vi "NML SCMPS make persistent.vi"(0 "VISA session":refnum<visa-resource-name>="GPIB0::22::INSTR") -> (2 "String":string, 3 "Persistent Field":dbl format="%.2f", 4 "Persistence Out":bool=TRUE)   [LabVIEW 2020]
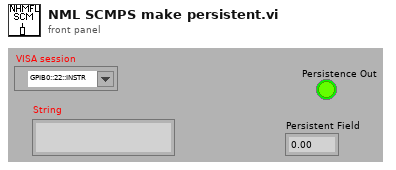
[diagram p1: front panel]
types:
  T1 = enum16{"No Response", "Ramping to programmed field ", "Holding at programmed field", "Paused", "Ramp Manual Up", "Ramp Manual Down", "Ramping to Zero", "QUENCH", "Heating Persistence Switch", "At Zero Current"}
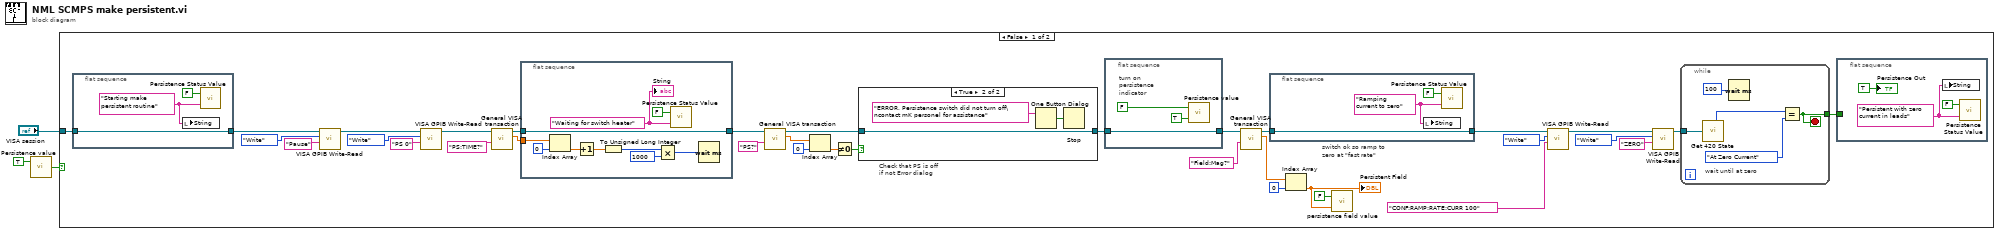
[diagram p0: block diagram]
diagram:
  n1 = call "Persistence value.vi"("Read/Write this vi"=TRUE ("Read/Write")) -> ("Persistence Out"=w2:bool)  [unwired: 1 in]
  n2 = case shown="False" w2 {
    tunnel: "VISA session" -> [w5 _]
    frame False {
      # "Check that PS is off \nif not Error dialog"
      # "switch ok so ramp to zero at \"fast rate\""
      n3 = flat-sequence {
        tunnel: w5 -> [w38]
        tunnel: [w38] -> w4
        frame #0 {
          w39 = "Starting make persistent routine"
          n4 = local write "String"(w39) -> ()
          n5 = call "Persistence Status Value.vi"("Persistence Status In"=w39, "Read/Write this vi"=FALSE) -> ()  [unwired: 1 out]
        }
      }
      n6 = call "VISA GPIB Write-Read.vi"("Command"="Pause" ("String to Write"), "Action"=enum16{"Write", "Read", "Write & Read"}."Write", "VISA resource name"=w4) -> ("dup VISA Session"=w12:refnum<visa-resource-name>)  [unwired: 5 in, 3 out]
      n7 = call "VISA GPIB Write-Read.vi"("Command"="PS 0" ("String to Write"), "Action"=enum16{"Write", "Read", "Write & Read"}."Write", "VISA resource name"=w12) -> ("dup VISA Session"=w17:refnum<visa-resource-name>)  [unwired: 5 in, 3 out]
      n8 = call "General VISA transaction.vi"("Command String"="PS:TIME?", "VISA Session"=w17) -> ("Measurement"=w15:dbl[], "dup VISA Session"=w16:refnum<visa-resource-name>)  [unwired: 4 in, 4 out]
      n9 = flat-sequence {
        tunnel: w16 -> [w41]
        tunnel: w15 -> [w42]
        tunnel: [w41] -> w19
        frame #0 {
          w50 = "Waiting for switch heater"
          n10 = Index Array(array=w42, index=0) -> (element=w45:dbl)
          n11 = Increment(x=w45) -> (x+1=w47:dbl)
          n12 = To Unsigned Long Integer(number=w47) -> (unsigned 32bit integer=w48:u32)
          n13 = Multiply(x=w48, y=u32 1000) -> (x*y=w46:u32)
          n14 = call "Persistence Status Value.vi"("Persistence Status In"=w50, "Read/Write this vi"=FALSE) -> ()  [unwired: 1 out]
          n15 = Wait (ms)(milliseconds to wait=w46) -> ()  [unwired: 1 out]
          "String" <- w50
        }
      }
      n16 = call "General VISA transaction.vi"("Command String"="PS?", "VISA Session"=w19) -> ("Measurement"=w24:dbl[], "dup VISA Session"=w20:refnum<visa-resource-name>)  [unwired: 4 in, 4 out]
      n17 = Index Array(array=w24, index=0) -> (element=w22:dbl)
      n18 = Not Equal To 0?(x=w22) -> (x != 0?=w21:bool)
      n19 = case shown="True" w21 {
        tunnel: w20 -> [w54 w55]
        tunnel: [w54 w55] -> w7
        frame False {
        }
        frame True {
          n20 = One Button Dialog(message="ERROR, Persistence switch did not turn off\ncontact mK personel for assistance") -> (true=w56:bool)  [unwired: 1 in]
          n21 = Stop(stop? (T)=w56) -> ()
        }
      }
      n22 = flat-sequence {
        tunnel: w7 -> [w51]
        tunnel: [w51] -> w6
        frame #0 {
          # "turn on persistence indicator"
          n23 = call "Persistence value.vi"("Persistence In"=TRUE, "Read/Write this vi"=FALSE) -> ()  [unwired: 1 out]
        }
      }
      n24 = call "General VISA transaction.vi"("Command String"="Field:Mag?", "VISA Session"=w6) -> ("Measurement"=w29:dbl[], "dup VISA Session"=w9:refnum<visa-resource-name>)  [unwired: 4 in, 4 out]
      n25 = flat-sequence {
        tunnel: w9 -> [w58]
        tunnel: [w58] -> w8
        frame #0 {
          w60 = "Ramping  current to zero" ("String")
          n26 = local write "String"(w60) -> ()
          n27 = call "Persistence Status Value.vi"("Persistence Status In"=w60, "Read/Write this vi"=FALSE) -> ()  [unwired: 1 out]
        }
      }
      n28 = Index Array(array=w29, index=0) -> (element=w27:dbl)
      "Persistent Field" <- w27
      n29 = call "persistence field value.vi"("Persistent Field In"=w27, "Read/Write this vi"=FALSE) -> ()  [unwired: 1 out]
      n30 = call "VISA GPIB Write-Read.vi"("Command"="CONF:RAMP:RATE:CURR 100" ("String to Write"), "Action"=enum16{"Write", "Read", "Write & Read"}."Write", "VISA resource name"=w8) -> ("dup VISA Session"=w33:refnum<visa-resource-name>)  [unwired: 5 in, 3 out]
      n31 = call "VISA GPIB Write-Read.vi"("Command"="ZERO" ("String to Write"), "Action"=enum16{"Write", "Read", "Write & Read"}."Write", "VISA resource name"=w33) -> ("dup VISA Session"=w36:refnum<visa-resource-name>)  [unwired: 5 in, 3 out]
      n32 = while {
        tunnel: w36 -> [w65]
        tunnel: [w61] -> w37
        stop <- w61 stop-if-true
        # "wait until at zero"
        n33 = call "Get 420 State.vi"("VISA session"=w65) -> ("State"=w64:T1)  [unwired: 5 out]
        n34 = Wait (ms)(milliseconds to wait=u32 100) -> ()  [unwired: 1 out]
        n35 = Equal?(x=w64, y=T1."At Zero Current") -> (x = y?=w61:bool)
      }
      n36 = flat-sequence {
        tunnel: w37 -> [_]
        frame #0 {
          w67 = "Persistent with zero current in leads" ("String")
          n37 = local write "String"(w67) -> ()
          n38 = call "Persistence Status Value.vi"("Persistence Status In"=w67, "Read/Write this vi"=FALSE) -> ()  [unwired: 1 out]
          "Persistence Out" <- TRUE
        }
      }
    }
    frame True {
      # "already persistent so skip the routine"
    }
  }
